vi "svacg_LimitTest Pass Scalar Limit.vi"(1 "In":dbl) -> (0 "Out":dbl)   [LabVIEW 2017]
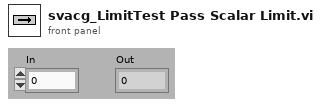
[diagram p1: front panel]
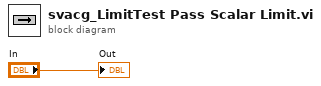
[diagram p0: block diagram]
diagram:
  "Out" <- "In"
